vi "configLockin.vi"(8 "error in (no error)":errorcluster, 11 "Channels: Lockin in":T1 {"REF phi (deg)" format="%#_3g"}) -> (0 "error out":errorcluster, 3 "Channels: Lockin out":T1 {"REF phi (deg)" format="%#_3g"})   [LabVIEW 2016]
uses:
  Typedefs/REF-cluster.ctl
  Typedefs/REF_f-array.ctl
  Typedefs/REF_phi-array.ctl
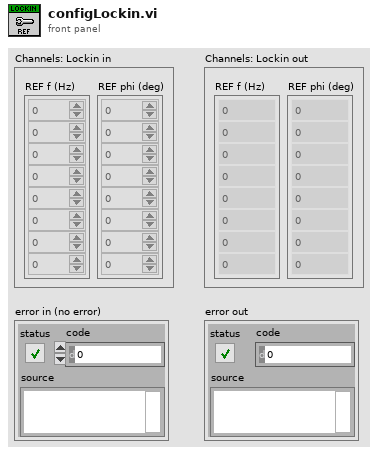
[diagram p1: front panel]
types:
  T1 = typedef "REF-cluster.ctl" = cluster{"REF f (Hz)":T2, "REF phi (deg)":T3}
  T2 = typedef "REF_f-array.ctl" = dbl[]
  T3 = typedef "REF_phi-array.ctl" = dbl[]
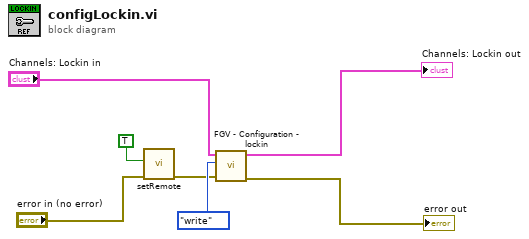
[diagram p0: block diagram]
diagram:
  n1 = call "setRemote.vi"("error in (no error)"="error in (no error)", "Remote Mode"=TRUE ("IV mode")) -> ("error out"=w2:errorcluster)  [unwired: 7 in]
  n2 = call "FGV - Configuration - lockin.vi"("error in"=w2, "Function"=enum16{"write", "read"}."write", "Channels: Lockin"="Channels: Lockin in") -> ("error out"=→"error out":errorcluster, "Channels: Lockin 2"=→"Channels: Lockin out":T1)  [unwired: 3 in]
